vi "Untitled 2.vi"() -> ()   [LabVIEW 2011]
uses:
  JSON Value/JSON Value.lvclass
  Variant JSON/Variant JSON.lvlib
panel:
  out "Time 2":dbl format="%#_6p"
  out "offset":i32
  in  "Numeric":dbl=10000.0
  in  "Type":bool
  out "Time":dbl format="%#_6p"
  out "JSON Value out":refnum<class "JSON Value.lvclass">
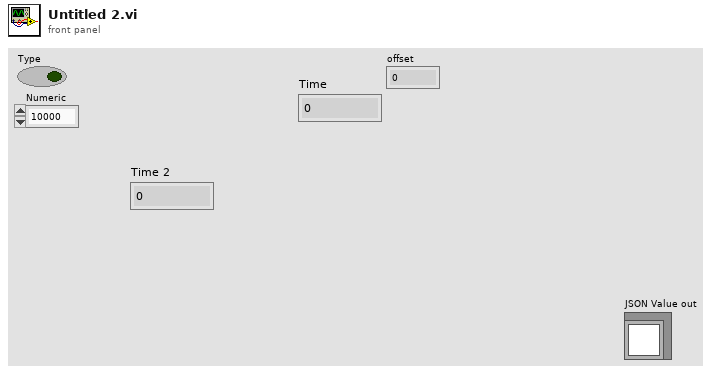
[diagram p1: front panel]
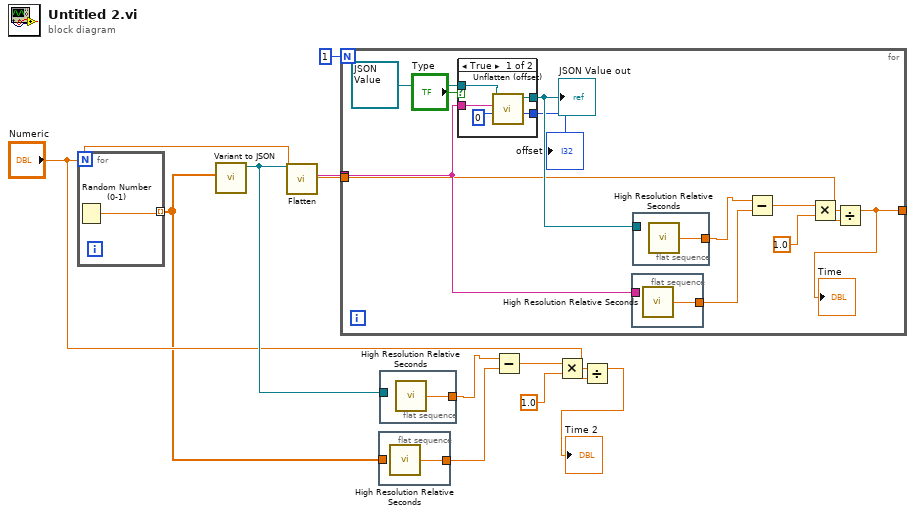
[diagram p0: block diagram]
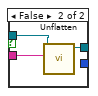
[diagram p2: hidden frame]
diagram:
  n1 = for {
    N: "Numeric" -> [_]
    tunnel: [w12] -> w1 mode=indexing
    n2 = Random Number (0-1)() -> (number: 0 to 1=w12:dbl)
  }
  n3 = call "Variant to JSON.vi"("Variant"=w1) -> ("JSON Value out"=w3:refnum<class "JSON Value.lvclass">)  [unwired: 9 in, 1 out]
  n4 = call-dynamic "Flatten.vi"("JSON Value in"=w3) -> ("String"=w4:string)  [unwired: 9 in, 1 out]
  n5 = for {
    N: 1 -> [_]
    tunnel: w4 -> [w22]
    tunnel: [w13] -> _
    tunnel: "Numeric" -> [w16]
    n6 = case shown="True" "Type" {
      tunnel: refnum<class "JSON Value.lvclass"> refnum ("JSON Value.lvclass") -> [w28 w32]
      tunnel: [w27 w31] -> w23
      tunnel: w22 -> [w26 w30]
      tunnel: [w25 _] -> w14
      frame True {
        n7 = call-dynamic "Unflatten (offset).vi"("offset (0)"=0, "JSON stream"=w26, "JSON Value in"=w28) -> ("offset"=w25:i32, "JSON Value out"=w27:refnum<class "JSON Value.lvclass">)  [unwired: 5 in, 2 out]
      }
      frame False {
        n8 = call-dynamic "Unflatten.vi"("JSON stream"=w30, "JSON Value in"=w32) -> ("JSON Value out"=w31:refnum<class "JSON Value.lvclass">)  [unwired: 6 in, 3 out]
      }
    }
    "JSON Value out" <- w23
    "offset" <- w14
    n9 = flat-sequence {
      tunnel: [w33] -> w17
      tunnel: w22 -> [_]
      frame #0 {
        n10 = call <vilib>:"High Resolution Relative Seconds.vi"() -> ("relative seconds"=w33:dbl)
      }
    }
    n11 = flat-sequence {
      tunnel: [w34] -> w18
      tunnel: w23 -> [_]
      frame #0 {
        n12 = call <vilib>:"High Resolution Relative Seconds.vi"() -> ("relative seconds"=w34:dbl)
      }
    }
    n13 = Subtract(x=w18, y=w17) -> (x-y=w20:dbl)
    n14 = Multiply(x=w20, y=1.0) -> (x*y=w21:dbl)
    n15 = Divide(x=w21, y=w16) -> (x/y=w13:dbl)
    "Time" <- w13
  }
  n16 = flat-sequence {
    tunnel: [w35] -> w9
    tunnel: w1 -> [_]
    frame #0 {
      n17 = call <vilib>:"High Resolution Relative Seconds.vi"() -> ("relative seconds"=w35:dbl)
    }
  }
  n18 = flat-sequence {
    tunnel: [w36] -> w8
    tunnel: w3 -> [_]
    frame #0 {
      n19 = call <vilib>:"High Resolution Relative Seconds.vi"() -> ("relative seconds"=w36:dbl)
    }
  }
  n20 = Subtract(x=w8, y=w9) -> (x-y=w6:dbl)
  n21 = Multiply(x=w6, y=1.0) -> (x*y=w5:dbl)
  n22 = Divide(x=w5, y="Numeric") -> (x/y=→"Time 2":dbl)
